vi "Authorization Kill License.vi"(8 "error in (no error)":errorcluster) -> (0 "error out":errorcluster)   [LabVIEW 2011]
doc: "The KillLicense() function is used to disable an existing license and provides a confirmation code that can be entered into the Site Key Generator in order to display the details of the de-authorization.\n\n0 Function was performed successfully.\n-1 CrypKey has not yet been initialized.\n-2 The protected program is not authorized\n-3 The license files are currently write protected.\n\nThe confirmation code provided by this function can be entered in the Site Code field of the Site Key Generator. Information about the license that was terminated is displayed when the \"check\" button is pressed.\n\n\nThis function does not remove the special hard-drive signature of the automatic licensing functions."
uses:
  Authorization Data.ctl
  Authorization Global.vi
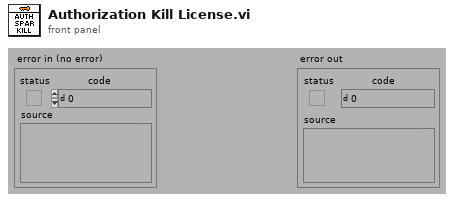
[diagram p1: front panel]
types:
  T1 = typedef "Authorization Data.ctl" = cluster{"Valid":bool, "Seats":i32, "Expire Time":timestamp, "Last Access Time":timestamp, "Product ID":string, "Hardware ID":string, "Spartan Serial Number":string, "Feature":cluster{"#attributes":cluster{"Name":string, "Value":string}}[]}
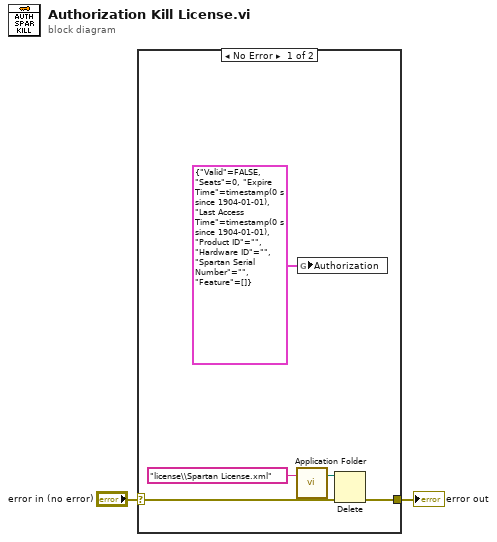
[diagram p0: block diagram]
diagram:
  n1 = case shown="No Error" "error in (no error)" {
    selector: "error in (no error)" -> [w6 w8]
    tunnel: [w5 w8] -> w1
    frame No Error {
      n2 = call "Application Folder.vi"("Relative Path (\"\" - Folder)"="license\\Spartan License.xml" ("regular expression")) -> ("Application Folder"=w4:path)  [unwired: 2 in]
      n3 = global write "Authorization Global.vi" "Authorization"(T1 {"Valid"=FALSE, "Seats"=0, "Expire Time"=timestamp(0 s since 1904-01-01), "Last Access Time"=timestamp(0 s since 1904-01-01), "Product ID"="", "Hardware ID"="", "Spartan Serial Number"="", "Feature"=[]} ("Authorization")) -> ()
      n4 = Delete(path (use dialog)=w4, error in=w6) -> (error out=w5:errorcluster)  [unwired: 3 in, 2 out]
    }
    frame Error {
    }
  }
  "error out" <- w1
